vi "sub_vacuum_main.vi"(8 "error in":errorcluster caption="에러 입력(에러 없음)") -> (0 "error out":errorcluster caption="에러 출력")   [LabVIEW 2013]
uses:
  ctl/UI_cmd-ctl.ctl
  <vilib>/Analysis/baseanly.llb/Mean (DBL).vi
  Global.vi
  <vilib>/Analysis/NI_AALPro.lvlib
  <vilib>/Analysis/NI_AALBase.lvlib
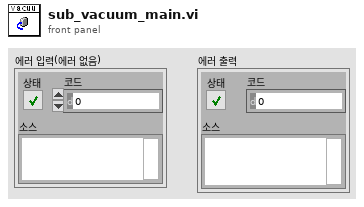
[diagram p1: front panel]
types:
  T1 = typedef "UI_cmd-ctl.ctl" = enum16{"default", "create", "read"}
  T2 = typedef "UI_ctl.ctl" = cluster{"Heater temp":refnum<vi>, "heater":refnum<vi>, "vacuum (kpa)":refnum<vi>, "Balance xy graph":refnum<vi>, "Strain chart w cal":refnum<vi>, "Pickup force":refnum<vi>, "Pickup time":refnum<vi>, "Data chart":refnum<vi>, "Trigger graph":refnum<vi>, "vacuum 차트":refnum<vi>, "vacuum":refnum<vi>, "Strain raw graph":refnum<vi>, "Strain raw chart":refnum<vi>, "Bonding time":refnum<vi>, "Bonding force":refnum<vi>, "Balance":refnum<vi>, "Filtered force graph":refnum<vi>, "ROI intensity":refnum<vi>, "Heater_rt":refnum<vi>, "Tensile force":refnum<vi>, "Force rt":refnum<vi>}
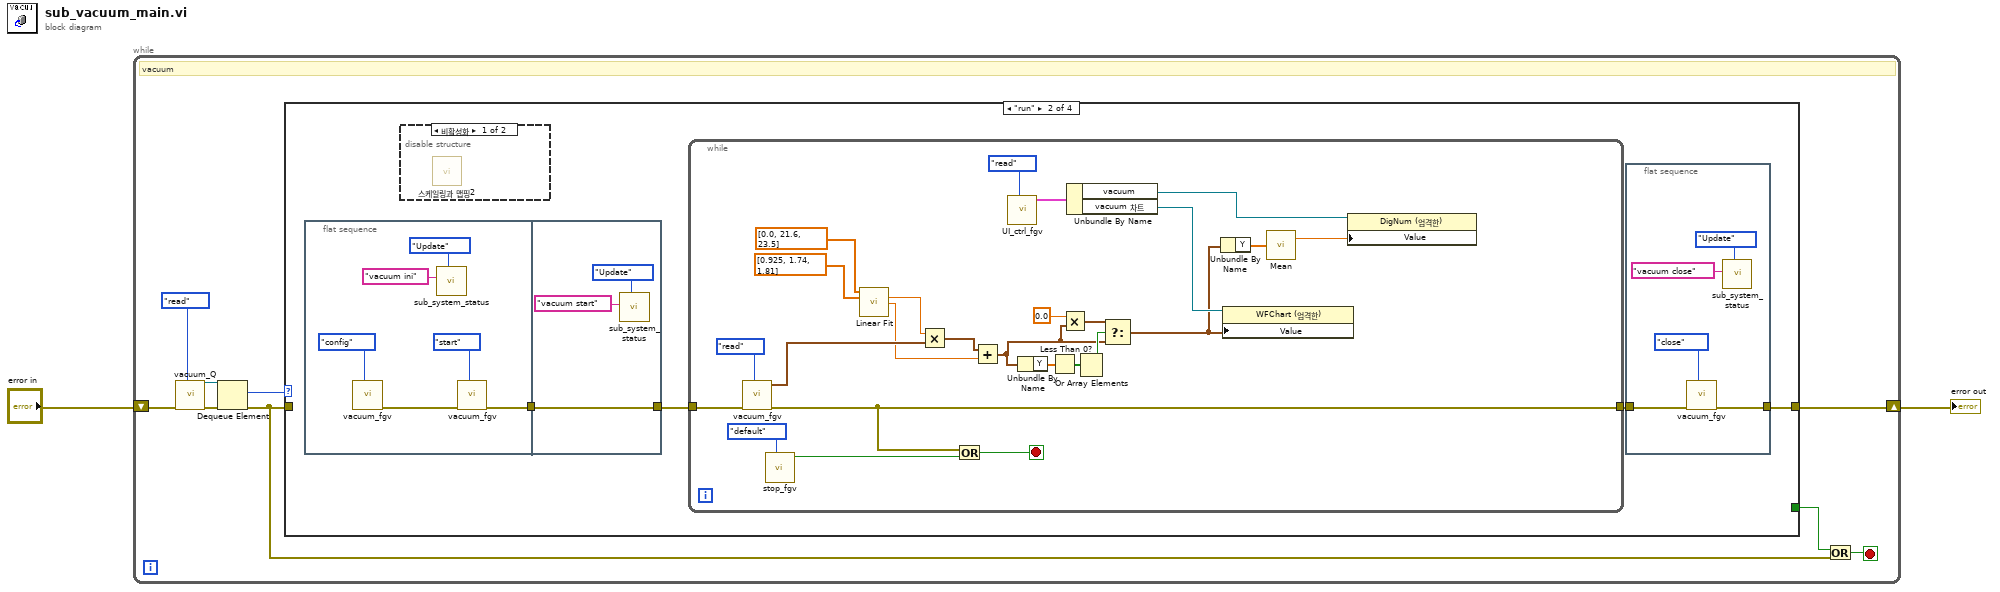
[diagram p0: block diagram]
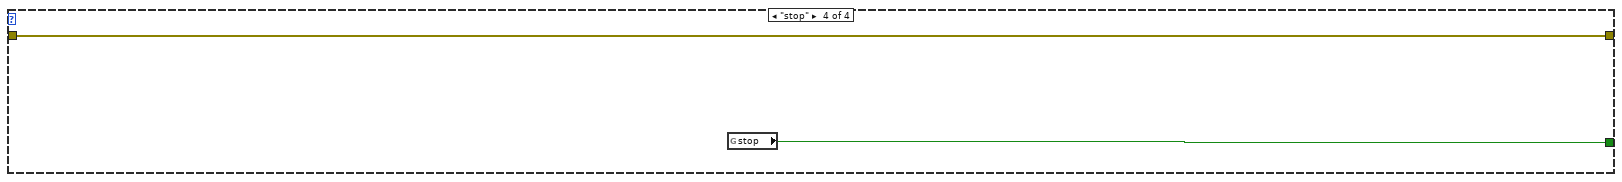
[diagram p5: hidden frame]
diagram:
  n1 = while {
    shift-right: [w5] -> w2
    shift-left: "error in" -> [w4]
    stop <- w7 stop-if-true
    # "vacuum"
    n2 = call "vacuum_Q.vi"("cmd"=enum16{"create", "write", "read", "close"}."read", "error in"=w4) -> ("error out"=w10:errorcluster, "queue out"=w9:refnum<queue>)  [unwired: 8 in]
    n3 = Dequeue Element(queue=w9, error in (no error)=w10) -> (element=w6:enum16{"config", "run", "pause", "stop"}, error out=w3:errorcluster)  [unwired: 1 in, 2 out]
    n4 = case shown="\"run\"" w6 {
      tunnel: [_ _ _ w58] -> w8
      tunnel: [w12 w14 w56 w57] -> w5
      tunnel: w3 -> [w12 _ w56 w57]
      frame "config", Default {
      }
      frame "run" {
        n5 = flat-sequence {
          tunnel: [w26] -> w13
          tunnel: [w30] -> w16
          tunnel: w13 -> [w30]
          frame #0 {
            n6 = call "vacuum_fgv.vi"("cmd"=enum16{"config", "start", "read", "close"}."config") -> ("error out"=w27:errorcluster)  [unwired: 9 in, 1 out]
            n7 = call "sub_system_status.vi"("Mode"=enum16{"Initial", "Update", "Clear"}."Update", "String in"="vacuum ini") -> ()  [unwired: 9 in, 1 out]
            n8 = call "vacuum_fgv.vi"("cmd"=enum16{"config", "start", "read", "close"}."start", "error in (no error)"=w27) -> ("error out"=w26:errorcluster)  [unwired: 8 in, 1 out]
          }
          frame #1 {
            n9 = call "sub_system_status.vi"("Mode"=enum16{"Initial", "Update", "Clear"}."Update", "String in"="vacuum start") -> ()  [unwired: 9 in, 1 out]
          }
        }
        n10 = disable-structure shown="비활성화" {
          frame Disabled {
            n11 = call "스케일링과 맵핑2"() -> ()  [unwired: 10 in, 2 out]
          }
          frame Enabled {
          }
        }
        n12 = while {
          tunnel: w16 -> [w53]
          tunnel: [w52] -> w15
          stop <- w50 stop-if-true
          n13 = call "vacuum_fgv.vi"("cmd"=enum16{"config", "start", "read", "close"}."read", "error in (no error)"=w53) -> ("error out"=w52:errorcluster, "data"=w45:waveform(dbl))  [unwired: 8 in]
          n14 = call "stop_fgv.vi"("cmd"=enum16{"default", "ini", "stop"}."default") -> ("stop"=w51:bool)  [unwired: 9 in, 1 out]
          n15 = call <vilib>:"Linear Fit.vi"("Y"=dbl[] [0.0, 21.6, 23.5] ("X"), "X"=dbl[] [0.925, 1.74, 1.81]) -> ("slope"=w42:dbl, "intercept"=w40:dbl)  [unwired: 9 in, 3 out]
          n16 = Multiply(x=w42, y=w45) -> (x*y=w41:waveform(dbl))
          n17 = Or(x=w52, y=w51) -> (x .or. y?=w50:bool)
          n18 = Add(x=w41, y=w40) -> (x+y=w35:waveform(dbl))
          n19 = call "UI_ctrl_fgv.vi"("cmd"=UI_cmd-ctl."read") -> ("UI cluster out"=w49:T2)  [unwired: 10 in]
          n20 = Unbundle By Name(w35) -> ("Y"=w39:dbl[])
          n21 = Less Than 0?(x=w39) -> (x < 0?=w38:bool[])
          n22 = Multiply(x=0.0, y=w35) -> (x*y=w36:waveform(dbl))
          n23 = Unbundle By Name(w49) -> ("vacuum"=w47:refnum<vi>, "vacuum 차트"=w48:refnum<vi>)
          n24 = Or Array Elements(Boolean array=w38) -> (logical OR=w37:bool)
          n25 = Select(t=w36, s=w37, f=w35) -> (s? t:f=w33:waveform(dbl))
          n26 = Unbundle By Name(w33) -> ("Y"=w32:dbl[])
          n27 = property class="WFChart (엄격한)"(reference=w48, "Value"=w33) -> ()  [unwired: 1 in, 2 out]
          n28 = call-poly <vilib>:"Mean.vi"("X"=w32) -> ("mean"=w31:dbl)  [unwired: 1 out]
          n29 = property class="DigNum (엄격한)"(reference=w47, "Value"=w31) -> ()  [unwired: 1 in, 2 out]
        }
        n30 = flat-sequence {
          tunnel: w15 -> [w21]
          tunnel: [w20] -> w14
          frame #0 {
            n31 = call "vacuum_fgv.vi"("cmd"=enum16{"config", "start", "read", "close"}."close", "error in (no error)"=w21) -> ("error out"=w20:errorcluster)  [unwired: 8 in, 1 out]
            n32 = call "sub_system_status.vi"("Mode"=enum16{"Initial", "Update", "Clear"}."Update", "String in"="vacuum close") -> ()  [unwired: 9 in, 1 out]
          }
        }
      }
      frame "pause" {
      }
      frame "stop" {
        n33 = global read "Global.vi" "stop"() -> (w58:bool)
      }
    }
    n34 = Or(x=w8, y=w3) -> (x .or. y?=w7:bool)
  }
  "error out" <- w2
